vi "PathPlanner_Trajectory_GeneratePath.vi"(8 "Reversed":bool, 9 "MaxAccel":dbl, 10 "MaxVel":dbl, 11 "PathPoints":T6[](array[typedef]) {"HolonomicRotation"."SIN" format="%13.4f"; "HolonomicRotation"."COS" format="%13.4f"; "HolonomicRotation"."VALUE" format="%13.4f"; "NextControl"."Y" format="%14.3f"; "NextControl"."X" format="%14.3f"; "PrevControl"."Y" format="%14.3f"; "PrevControl"."X" format="%14.3f"; "AnchorPoint"."Y" format="%14.3f"; "AnchorPoint"."X" format="%14.3f"}) -> (3 "PathPlannerStates":T1[](array[typedef]) {"HolonomicAngular\nvelocity Deg/Sec"."SIN" format="%13.4f"; "HolonomicAngular\nvelocity Deg/Sec"."COS" format="%13.4f"; "HolonomicAngular\nvelocity Deg/Sec"."VALUE" format="%13.4f"; "HolonomicRotation"."SIN" format="%13.4f"; "HolonomicRotation"."COS" format="%13.4f"; "HolonomicRotation"."VALUE" format="%13.4f"; "AngularVelocity"."SIN" format="%13.4f"; "AngularVelocity"."COS" format="%13.4f"; "AngularVelocity"."VALUE" format="%13.4f"; "TrajectoryState"."POSE"."ROTATION"."SIN" format="%13.4f"; "TrajectoryState"."POSE"."ROTATION"."COS" format="%13.4f"; "TrajectoryState"."POSE"."ROTATION"."VALUE" format="%13.4f"; "TrajectoryState"."POSE"."TRANSLATION"."Y" format="%14.3f"; "TrajectoryState"."POSE"."TRANSLATION"."X" format="%14.3f"; "AngularAcceleration"."SIN" format="%13.4f"; "AngularAcceleration"."COS" format="%13.4f"; "AngularAcceleration"."VALUE" format="%13.4f"})   [LabVIEW 2019, in "PathPlanner.lvlib"]
uses:
  PathPlanner.lvlib
  PathPlannerWaypoint.ctl
  <vilib>/Rock Robotics/WPI/ThirdParty/JAS_Junk/TrajLib/TypeDef/TRANSLATION2D.ctl
  <vilib>/Rock Robotics/WPI/ThirdParty/JAS_Junk/TrajLib/TypeDef/ROTATION2D.ctl
  PathPlannerState.ctl
  <vilib>/Rock Robotics/WPI/ThirdParty/JAS_Junk/TrajLib/TypeDef/TRAJ_STATE.ctl
  <vilib>/Rock Robotics/WPI/ThirdParty/JAS_Junk/TrajLib/TypeDef/POSE2D.ctl
  <vilib>/Rock Robotics/WPI/ThirdParty/JAS_Junk/TrajLib/Trajectory_Library.lvlib
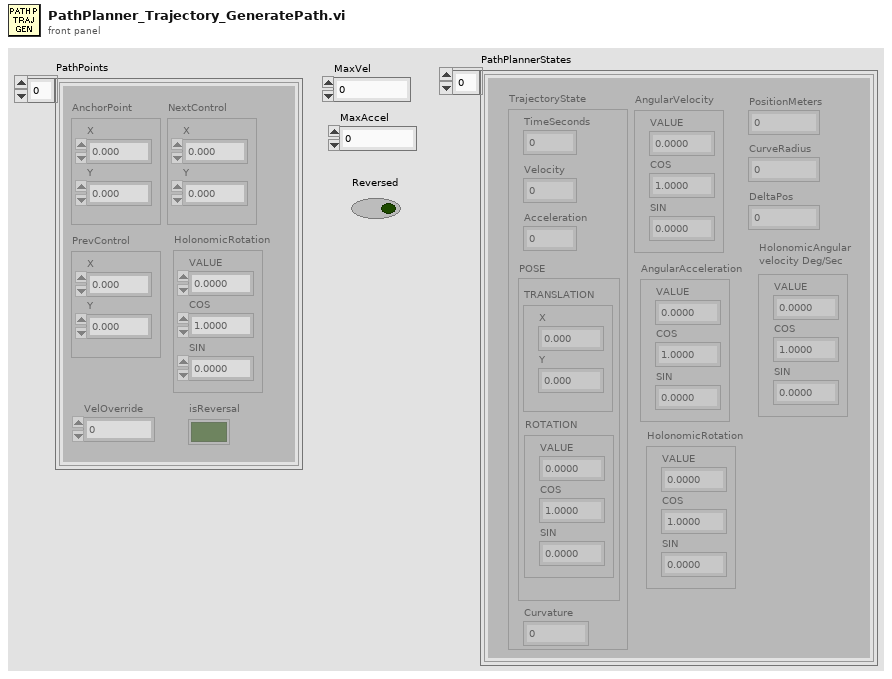
[diagram p1: front panel]
types:
  T1 = typedef "PathPlanner.lvlib/PathPlannerState.ctl" = cluster{"AngularAcceleration":T2, "PositionMeters":dbl, "TrajectoryState":T3, "AngularVelocity":T2, "HolonomicRotation":T2, "CurveRadius":dbl, "DeltaPos":dbl, "HolonomicAngular\nvelocity Deg/Sec":T2}
  T2 = typedef "Trajectory_Library.lvlib/ROTATION2D.ctl" = cluster{"VALUE":dbl, "COS":dbl, "SIN":dbl}
  T3 = typedef "Trajectory_Library.lvlib/TRAJ_STATE.ctl" = cluster{"TimeSeconds":dbl, "Velocity":dbl, "Acceleration":dbl, "POSE":T4, "Curvature":dbl}
  T4 = typedef "Trajectory_Library.lvlib/POSE2D.ctl" = cluster{"TRANSLATION":T5, "ROTATION":T2}
  T5 = typedef "Trajectory_Library.lvlib/TRANSLATION2D.ctl" = cluster{"X":dbl, "Y":dbl}
  T6 = typedef "PathPlanner.lvlib/PathPlannerWaypoint.ctl" = cluster{"AnchorPoint":T5, "PrevControl":T5, "NextControl":T5, "HolonomicRotation":T2, "VelOverride":dbl, "isReversal":bool}
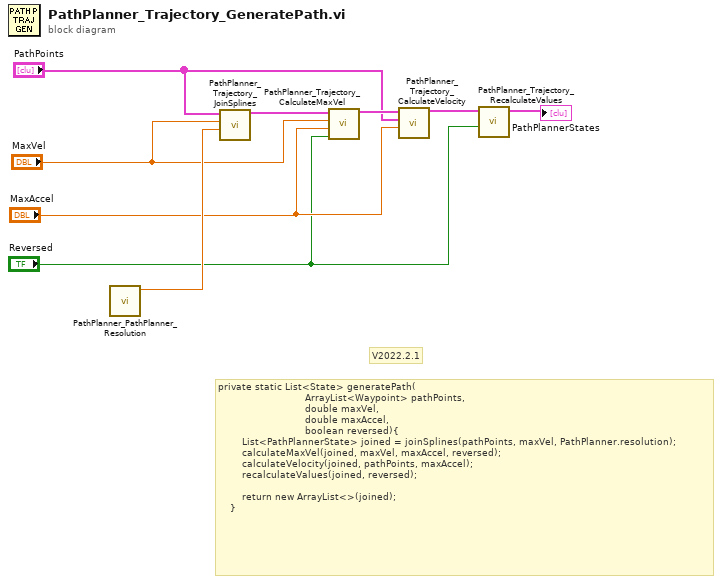
[diagram p0: block diagram]
diagram:
  # "private static List<State> generatePath(\n                             ArrayList<Waypoint> pathPoints, \n                             double maxVel, \n                             double maxAccel, \n                             boolean reversed){\n        List<PathPlannerState> joined = joinSplines(pathPoints, maxVel, PathPlanner.resolution);\n        calculateMaxVel(joined, maxVel, maxAccel, reversed);\n        calculateVelocity(joined, pathPoints, maxAccel);\n        recalculateValues(joined, reversed);\n\n        return new ArrayList<>(joined);\n    }"
  # "V2022.2.1"
  n1 = call "PathPlanner_PathPlanner_Resolution.vi"() -> ("Resolution"=w9:dbl)  [unwired: 11 in]
  n2 = call "PathPlanner_Trajectory_JoinSplines.vi"("Step"=w9, "Max Velocity"="MaxVel", "PathPoints"="PathPoints") -> ("outPathPlannerStates"=w8:T1[])  [unwired: 8 in]
  n3 = call "PathPlanner_Trajectory_CalculateMaxVel.vi"("Reversed"="Reversed", "MaxAccel"="MaxAccel", "MaxVel"="MaxVel", "PathPlannerStates"=w8) -> ("outPathPlannerStates"=w6:T1[])  [unwired: 7 in]
  n4 = call "PathPlanner_Trajectory_CalculateVelocity.vi"("MaxAccel"="MaxAccel", "PathPoints"="PathPoints", "PathPlannerStates"=w6) -> ("outPathPlannerStates"=w3:T1[])  [unwired: 8 in]
  n5 = call "PathPlanner_Trajectory_RecalculateValues.vi"("Reversed"="Reversed", "PathPlannerStates"=w3) -> ("outPathPlannerStates"=→"PathPlannerStates":T1[])  [unwired: 9 in]
